vi "ALTER HDG VECTOR.vi"(0 "Joystick angle (deg CCW)":dbl, 1 "drive frame":T2, 2 "front face":T3, 3 "Alliance":T1, 4 "ROBOT compass reading (deg CW)":dbl) -> (14 "Joystick (deg)":dbl)   [LabVIEW 2023]
uses:
  ctrl defs/ctrl FRONT FACE selector.ctl
  ctrl defs/ctrl DRIVING FRAME selector.ctl
  <vilib>/Rock Robotics/WPI/DriverStation/WPI_DriverStationAllianceInfo.ctl
  <vilib>/Analysis/coordinate.llb/Angle Units.ctl
  <vilib>/Analysis/coordinate.llb/Angle Range (Degree).ctl
  <vilib>/Analysis/coordinate.llb/Wrap Angle (scalar).vi
  Global odometry.vi
  <vilib>/Analysis/NI_AAL_Angle.lvlib
panel:
  out "error out":errorcluster
  in  "error in (no error)":errorcluster
  out "adjust for FRONT":dbl
  out "downfield\nmagnetic\nHDG (deg)":dbl
  out "robot angle wrt FRONT":dbl
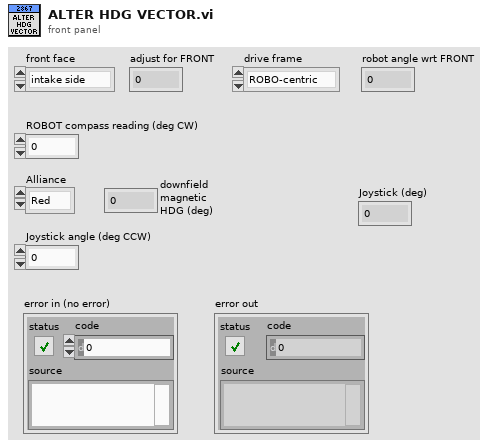
[diagram p1: front panel]
types:
  T1 = typedef "WPI_DriverStationAllianceInfo.ctl" = enum16{"Red", "Blue", "Invalid"}
  T2 = typedef "ctrl DRIVING FRAME selector.ctl" = enum16{"ROBO-centric", "FLD-centric"}
  T3 = typedef "ctrl FRONT FACE selector.ctl" = enum16{"intake side", "shooter side"}
  T4 = typedef "NI_AAL_Angle.lvlib/Angle Range (Degree).ctl" = u16
  T5 = typedef "NI_AAL_Angle.lvlib/Angle Units.ctl" = i32
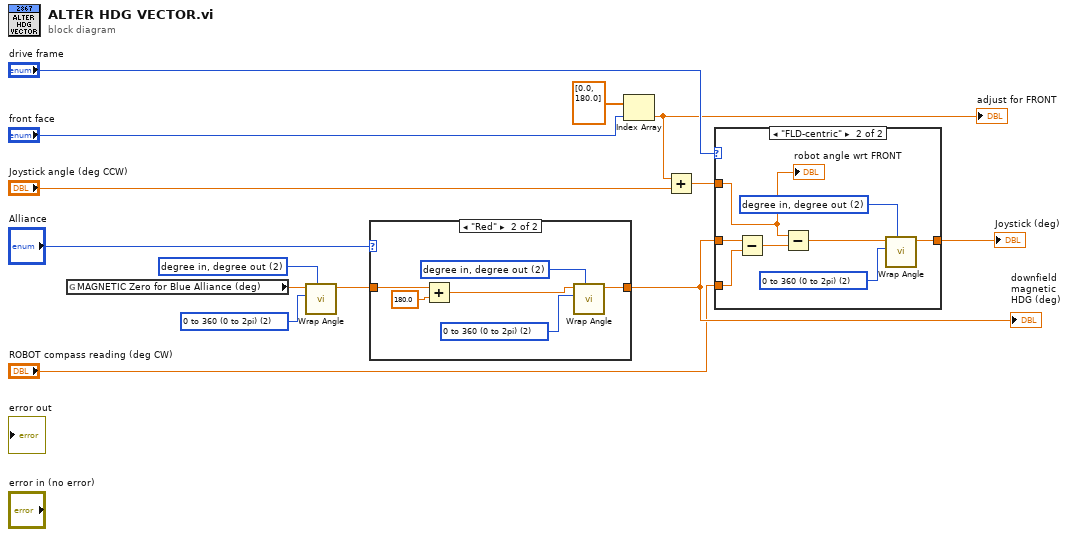
[diagram p0: block diagram]
diagram:
  w7 = T4 2 items=["none", "-180 to 180 (-pi to pi)", "0 to 360 (0 to 2pi)"] ("angle range")
  w6 = T5 2 items=["radian in, radian out", "radian in, degree out", "degree in, degree out", "degree in, radian out"] ("angle units")
  n1 = global read "Global odometry.vi" "MAGNETIC Zero for Blue Alliance (deg)"() -> (w4:dbl)
  n2 = call-poly <vilib>:"Wrap Angle.vi"("angle units"=w6, "angle range"=w7, "angle in"=w4) -> ("angle out"=w8:dbl)  [unwired: 7 in, 1 out]
  n3 = case shown="\"Red\"" "Alliance" {
    tunnel: w8 -> [w15 w21]
    tunnel: [w15 w18] -> w14
    frame "Blue", Default {
    }
    frame "Red" {
      w20 = T4 2 items=["none", "-180 to 180 (-pi to pi)", "0 to 360 (0 to 2pi)"] ("angle range")
      w19 = T5 2 items=["radian in, radian out", "radian in, degree out", "degree in, degree out", "degree in, radian out"] ("angle units")
      n4 = Add(x=w21, y=180.0) -> (x+y=w17:dbl)
      n5 = call-poly <vilib>:"Wrap Angle.vi"("angle units"=w19, "angle range"=w20, "angle in"=w17) -> ("angle out"=w18:dbl)  [unwired: 7 in, 1 out]
    }
  }
  "downfield\nmagnetic\nHDG (deg)" <- w14
  n6 = Index Array(array=dbl[] [0.0, 180.0], index="front face") -> (element=w3:dbl)
  "adjust for FRONT" <- w3
  n7 = Add(x=w3, y="Joystick angle (deg CCW)") -> (x+y=w11:dbl)
  n8 = case shown="\"FLD-centric\"" "drive frame" {
    tunnel: w11 -> [w22 w26]
    tunnel: [w22 w30] -> w10
    tunnel: "ROBOT compass reading (deg CW)" -> [_ w24]
    tunnel: w14 -> [_ w23]
    frame "ROBO-centric", Default {
    }
    frame "FLD-centric" {
      w28 = T5 2 items=["radian in, radian out", "radian in, degree out", "degree in, degree out", "degree in, radian out"] ("angle units")
      w29 = T4 2 items=["none", "-180 to 180 (-pi to pi)", "0 to 360 (0 to 2pi)"] ("angle range")
      n9 = Subtract(x=w23, y=w24) -> (x-y=w25:dbl)
      n10 = Subtract(x=w26, y=w25) -> (x-y=w27:dbl)
      n11 = call-poly <vilib>:"Wrap Angle.vi"("angle units"=w28, "angle range"=w29, "angle in"=w27) -> ("angle out"=w30:dbl)  [unwired: 7 in, 1 out]
      "robot angle wrt FRONT" <- w26
    }
  }
  "Joystick (deg)" <- w10
